vi "LocalSense_Powerstage_v1.vi"() -> (2 "Vline BC":dbl format="%#_8g", 3 "Vline AB":dbl format="%#_8g")   [LabVIEW 2022 SP3]
uses:
  Serial Board Com/Board Select.ctl
  Serial Board Com/ADCSelector BB.ctl
  HMP4000 Communication/HMP4040_ChannelControl.ctl
  <vilib>/DAQmx/write.llb/DAQmx Write (Digital 1D Bool NChan 1Samp 1Line).vi
  <vilib>/DAQmx/miscellaneous.llb/DAQmx Fill In Error Info.vi
panel:
  in  "error in (no error)":errorcluster
  out "Voltage Array":dbl[](array[numeric])
  out "error out":errorcluster
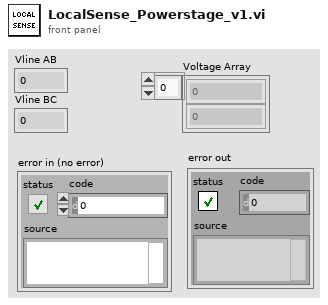
[diagram p1: front panel]
types:
  T1 = typedef "HMP4040_ChannelControl.ctl" = cluster{"CH1 Voltage":dbl, "CH1 Current":dbl, "CH1 Output":bool, "CH2 Voltage":dbl, "CH2 Current":dbl, "CH2 Output":bool, "CH3 Voltage":dbl, "CH3 Current":dbl, "CH3 Output":bool, "CH4 Voltage":dbl, "CH4 Current":dbl, "CH4 Output":bool, "Master Output":bool}
  T2 = typedef "ADCSelector BB.ctl" = enum16{"INVA_ISENSE_U", "INVA_ISENSE_V", "INVA_ISENSE_W", "INVA_UDC", "INVA_TEMP", "HB_TEMP", "AUXB_TEMP", "VLINE_AB", "VLINE_BC", "VLINE_CA", "VSENSE_POS_24V", "VSENSE_POS_5V", "VSENSE_NEG_15V", "INVB_ISENSE_U", "INV_B_ISENSEV", "INVB_ISENSE_W", "INVB_UDC", "INVB_TEMP", "AUXA_TEMP", "AUXC_TEMP", "VOUT_AB", "VOUT_BC", "VOUT_CA", "VSENSE_POS_15V", "VSENSE_POS_3P3V", "TEST_POINT"}
  T3 = typedef "Board Select.ctl" = enum16{"Blue Board", "Green Board"}
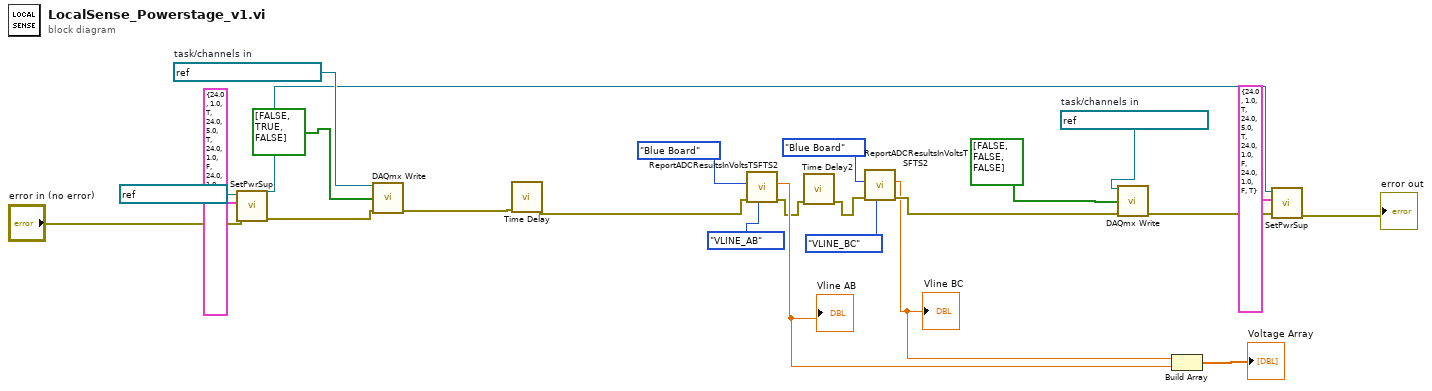
[diagram p0: block diagram]
diagram:
  w21 = refnum<k21> "FTS2_LocalSenseRelays"  # task/channels in
  w24 = refnum<k21> "FTS2_LocalSenseRelays"  # task/channels in
  n1 = call "SetPwrSup.vi"("error in (no error)"="error in (no error)", "HMP4040 Channel Settings"=T1 {"CH1 Voltage"=24.0, "CH1 Current"=1.0, "CH1 Output"=TRUE, "CH2 Voltage"=24.0, "CH2 Current"=5.0, "CH2 Output"=TRUE, "CH3 Voltage"=24.0, "CH3 Current"=1.0, "CH3 Output"=FALSE, "CH4 Voltage"=24.0, "CH4 Current"=1.0, "CH4 Output"=TRUE, "Master Output"=TRUE}, "HMP4040 IN"=refnum<visa-resource-name> "HMP4040_FTS2") -> ("error out"=w7:errorcluster, "HMP4040_OUT"=w2:refnum<visa-resource-name>)  [unwired: 7 in]
  n2 = call-poly <vilib>:"DAQmx Write.vi"("task/channels in"=w24, "data"=bool[] [FALSE, TRUE, FALSE], "error in"=w7) -> ("error out"=w20:errorcluster)  [unwired: 10 in, 2 out]
  n3 = call "Time Delay"("error in (no error)"=w20) -> ("error out"=w19:errorcluster)  [unwired: 10 in]
  n4 = call "ReportADCResultsInVoltsTSFTS2.vi"("Blue Board Enum"=ADCSelector_BB."VLINE_AB", "error in (no error)"=w19, "Board Selector"=Board_Select."Blue Board") -> ("error out"=w10:errorcluster, "Result"=w12:dbl)  [unwired: 5 in, 2 out]
  "Vline AB" <- w12
  n5 = call "Time Delay2"("error in (no error)"=w10) -> ("error out"=w9:errorcluster)  [unwired: 10 in]
  n6 = call "ReportADCResultsInVoltsTSFTS2.vi"("Blue Board Enum"=ADCSelector_BB."VLINE_BC", "error in (no error)"=w9, "Board Selector"=Board_Select."Blue Board") -> ("error out"=w16:errorcluster, "Result"=w11:dbl)  [unwired: 5 in, 2 out]
  "Vline BC" <- w11
  n7 = call-poly <vilib>:"DAQmx Write.vi"("task/channels in"=w21, "data"=bool[] [FALSE, FALSE, FALSE], "error in"=w16) -> ("error out"=w4:errorcluster)  [unwired: 10 in, 2 out]
  n8 = Build Array(w11, w12) -> (→"Voltage Array":dbl[])
  n9 = call "SetPwrSup.vi"("error in (no error)"=w4, "HMP4040 Channel Settings"=T1 {"CH1 Voltage"=24.0, "CH1 Current"=1.0, "CH1 Output"=TRUE, "CH2 Voltage"=24.0, "CH2 Current"=5.0, "CH2 Output"=TRUE, "CH3 Voltage"=24.0, "CH3 Current"=1.0, "CH3 Output"=FALSE, "CH4 Voltage"=24.0, "CH4 Current"=1.0, "CH4 Output"=FALSE, "Master Output"=TRUE}, "HMP4040 IN"=w2) -> ("error out"=→"error out":errorcluster)  [unwired: 7 in, 1 out]
